vi "Query (ObsReg).vi"(6 "timeout in ms (5000)":i32=5000, 8 "error in (no error)":errorcluster, 10 "Label":string, 11 "Send":refnum<class "Send.lvclass">) -> (0 "error out":errorcluster, 2 "Reply":refnum<class "MSG.lvclass">, 3 "Send":refnum<class "Send.lvclass">)   [LabVIEW 2011, in "Messenging.lvlib" / "ObserverRegistry.lvclass"]
uses:
  ObserverRegistry.lvclass
  Commands/Register by Label/Observer_RegisterByLabel.lvclass
  Interprocess Messenger/QueueMessenger/QueueMessenger.lvclass
  Interprocess Messenger/Send/Send.lvclass
  Interprocess Messenger/TextVarientMessage/MSG.lvclass
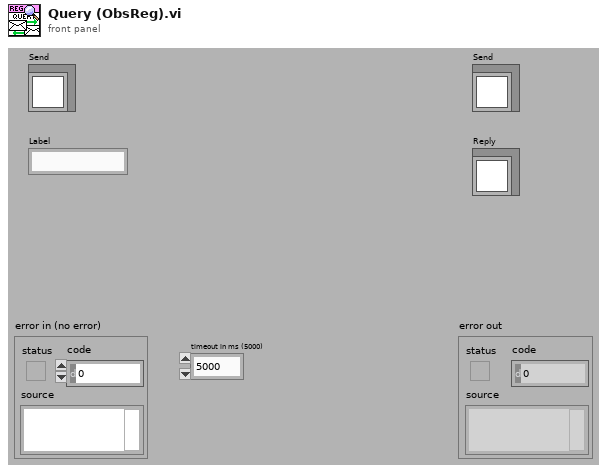
[diagram p1: front panel]
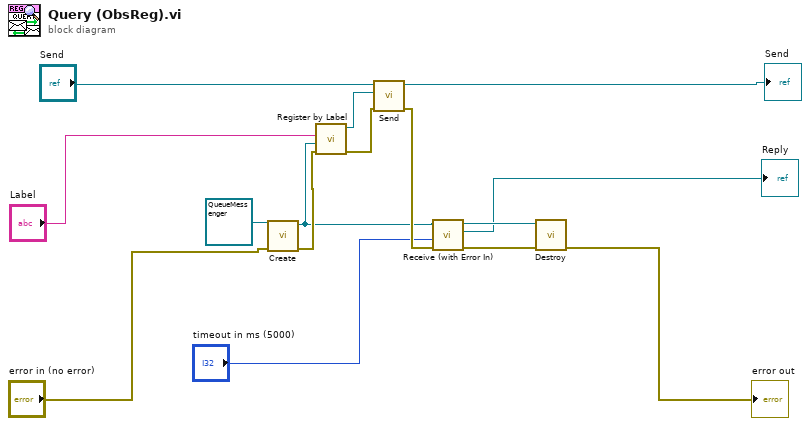
[diagram p0: block diagram]
diagram:
  n1 = call-dynamic "Create.vi"("error in (no error)"="error in (no error)", "QueueMessenger in"=refnum<class "QueueMessenger.lvclass"> refnum ("QueueMessenger.lvclass")) -> ("error out"=w8:errorcluster, "QueueMessenger out"=w5:refnum<class "QueueMessenger.lvclass">)  [unwired: 8 out]
  n2 = call "Register by Label.vi"("error in (no error)"=w8, "Observer"=w5, "Label to Register For"="Label") -> ("error out"=w7:errorcluster, "ObserverRegistryCommand_RegisterByLabel out"=w6:refnum<class "Observer_RegisterByLabel.lvclass">)  [unwired: 7 out]
  n3 = call-dynamic "Send.vi"("error in (no error)"=w7, "Message"=w6, "MSR Parent in"="Send") -> ("error out"=w12:errorcluster, "MSR Parent out"=→"Send":refnum<class "Send.lvclass">)  [unwired: 7 out]
  n4 = call-dynamic "Receive (with Error In).vi"("error in (no error)"=w12, "timeout in ms (5000)"="timeout in ms (5000)", "MGR in"=w5) -> ("error out"=w15:errorcluster, "Message"=→"Reply":refnum<class "MSG.lvclass">, "MGR out"=w14:refnum<class "QueueMessenger.lvclass">)  [unwired: 6 out]
  n5 = call-dynamic "Destroy.vi"("error in (no error)"=w15, "QueueMessenger in"=w14) -> ("error out"=→"error out":errorcluster)  [unwired: 9 out]
